vi "Create Sensor File.vi"(8 "error in (no error)":errorcluster, 10 "Item Configurations":refnum<class "Item Configuration.lvclass">[](array[class]), 11 "Top Level Path":path) -> (0 "error out":errorcluster)   [LabVIEW 2013, in "File IO.lvlib"]
uses:
  File IO.lvlib
  Item Configuration/Item Configuration/Item Configuration.lvclass
  <vilib>/xml/Load XML String.vi
  <vilib>/xml/Close Reference(Node).vi
  <vilib>/xml/NI_XML.lvlib
  <resource>/objmgr/DOMUserDefRef.rc
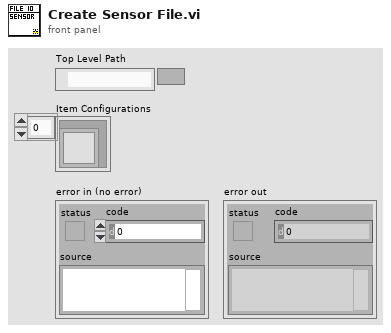
[diagram p1: front panel]
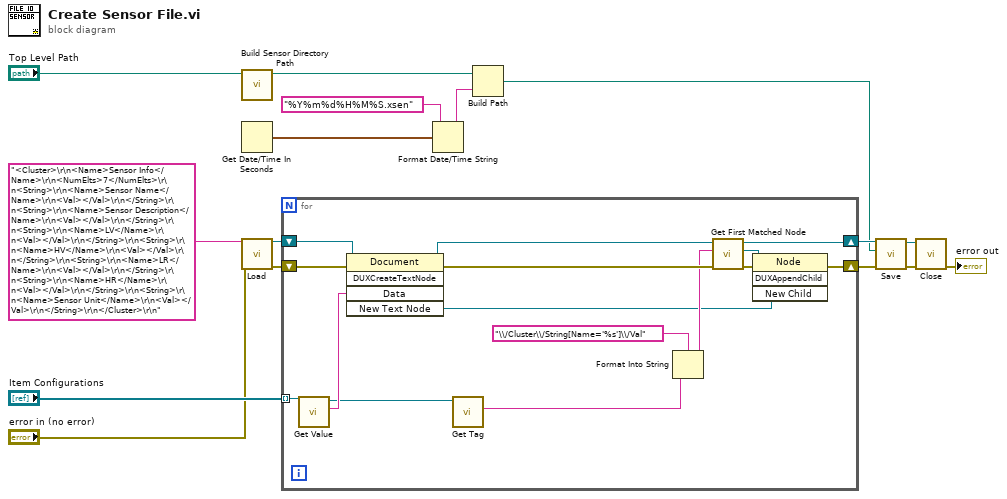
[diagram p0: block diagram]
diagram:
  n1 = call "Build Sensor Directory Path.vi"("Top Level Path"="Top Level Path") -> ("Sensor Directory Path"=w4:path)  [unwired: 10 in]
  n2 = Get Date/Time In Seconds() -> (seconds since 1Jan1904=w3:timestamp)
  n3 = call-poly <vilib>:"Load.vi"("XML string"="<Cluster>\r\n<Name>Sensor Info</Name>\r\n<NumElts>7</NumElts>\r\n<String>\r\n<Name>Sensor Name</Name>\r\n<Val></Val>\r\n</String>\r\n<String>\r\n<Name>Sensor Description</Name>\r\n<Val></Val>\r\n</String>\r\n<String>\r\n<Name>LV</Name>\r\n<Val></Val>\r\n</String>\r\n<String>\r\n<Name>HV</Name>\r\n<Val></Val>\r\n</String>\r\n<String>\r\n<Name>LR</Name>\r\n<Val></Val>\r\n</String>\r\n<String>\r\n<Name>HR</Name>\r\n<Val></Val>\r\n</String>\r\n<String>\r\n<Name>Sensor Unit</Name>\r\n<Val></Val>\r\n</String>\r\n</Cluster>\r\n" ("xml string"), "error in (no error)"="error in (no error)") -> ("DOM document out"=w16:refnum<k20>, "error out"=w15:errorcluster)  [unwired: 11 in, 1 out]
  n4 = for {
    shift-right: [w31] -> w12
    shift-left: w16 -> [w28]
    shift-right: [w24] -> w11
    shift-left: w15 -> [w27]
    tunnel: "Item Configurations" -> [w23] mode=indexing
    n5 = call-dynamic "Get Value.vi"("Item Configuration in"=w23) -> ("Project Info Value"=w22:string, "Item Configuration out"=w19:refnum<class "Item Configuration.lvclass">)  [unwired: 8 in, 1 out]
    n6 = invoke class="Document" method="DUXCreateTextNode"(reference=w28, error in=w27, "Data"=w22) -> (reference out=w29:refnum<k20>, error out=w26:errorcluster, "New Text Node"=w17:refnum<k20>)  [unwired: 2 in, 2 out]
    n7 = call-dynamic "Get Tag.vi"("Item Configuration in"=w19) -> ("Project Info Tag"=w20:string)  [unwired: 8 in, 2 out]
    n8 = Format Into String(format string="\\/Cluster\\/String[Name='%s']\\/Val" ("XPath expression"), w20) -> (resulting string=w18:string)  [unwired: 2 in, 1 out]
    n9 = call <vilib>:"Get First Matched Node.vi"("error in (no error)"=w26, "XPath expression"=w18, "node in"=w29) -> ("error out"=w25:errorcluster, "node result"=w30:refnum<k20>, "node out"=w31:refnum<k20>)  [unwired: 6 in]
    n10 = invoke class="Node" method="DUXAppendChild"(reference=w30, error in=w25, "New Child"=w17) -> (error out=w24:errorcluster)  [unwired: 1 in, 3 out]
  }
  n11 = Format Date/Time String(time format string (%c)="%Y%m%d%H%M%S.xsen", seconds (now)=w3) -> (date/time string=w2:string)  [unwired: 1 in]
  n12 = Build Path(base path=w4, name or relative path=w2) -> (appended path=w1:path)
  n13 = call <vilib>:"Save.vi"("error in (no error)"=w11, "XML file path"=w1, "DOM document in"=w12) -> ("error out"=w9:errorcluster, "DOM document out"=w10:refnum<k20>)  [unwired: 6 in, 1 out]
  n14 = call-poly <vilib>:"Close.vi"("error in (no error)"=w9, "node"=w10) -> ("error out"=→"error out":errorcluster)  [unwired: 7 in]
